vi "Smile_Or_Frown.vi"() -> (0 "New Values In":string[][](array[string])=[["Test data5"]], 1 "New Chs In":string[](array[string])=["30-10-03:New:Channel new5"])   [LabVIEW 2022 SP3]
uses:
  <vilib>/Analysis/baseanly.llb/Mean (DBL).vi
  Results_plotter_Global.vi
  Data plotting/subVIs/Plot_Values_Global.vi
  <vilib>/Analysis/NI_AALBase.lvlib
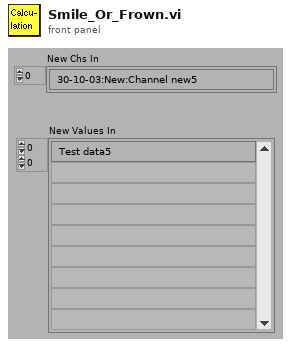
[diagram p1: front panel]
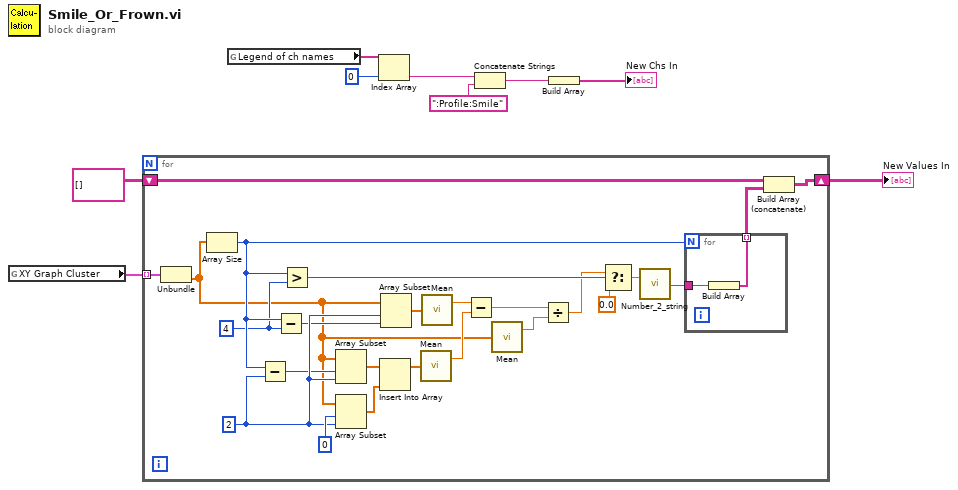
[diagram p0: block diagram]
diagram:
  n1 = global read "Plot_Values_Global.vi" "XY Graph Cluster"() -> (w1:cluster{dbl[], dbl[]}[])
  n2 = for {
    tunnel: w1 -> [w33] mode=indexing
    shift-right: [w30] -> w5
    shift-left: string[][] [] -> [w32]
    w22 = 2 ("length")
    w16 = 4 ("y")
    n3 = Unbundle(w33) -> (w13:dbl[])  [unwired: 1 out]
    n4 = Array Size(array=w13) -> (size(s)=w17:i32)
    n5 = Subtract(x=w17, y=w22) -> (x-y=w15:i32)
    n6 = Subtract(x=w17, y=w16) -> (x-y=w14:i32)
    n7 = Greater?(x=w17, y=w16) -> (0:w20:bool)
    n8 = Array Subset(array=w13, index=w15, length=w22) -> (w27:dbl[])
    n9 = Array Subset(array=w13, index=0, length=w22) -> (w26:dbl[])
    n10 = Insert Into Array(array=w27, new element=w26) -> (w25:dbl[])  [unwired: 1 in]
    n11 = Array Subset(array=w13, index=w22, length=w14) -> (w21:dbl[])
    n12 = call-poly <vilib>:"Mean.vi"("X"=w25) -> ("mean"=w23:dbl)  [unwired: 1 out]
    n13 = call-poly <vilib>:"Mean.vi"("X"=w21) -> ("mean"=w24:dbl)  [unwired: 1 out]
    n14 = Subtract(x=w24, y=w23) -> (x-y=w11:dbl)
    n15 = call-poly <vilib>:"Mean.vi"("X"=w13) -> ("mean"=w12:dbl)  [unwired: 1 out]
    n16 = Divide(x=w11, y=w12) -> (x/y=w10:dbl)
    n17 = Select(t=w10, s=w20, f=0.0) -> (s? t:f=w18:dbl)
    n18 = call "Number_2_string.vi"("number"=w18) -> ("String"=w29:string)  [unwired: 1 in]
    n19 = for {
      N: w17 -> [_]
      tunnel: [w35] -> w31 mode=indexing
      tunnel: w29 -> [w34]
      n20 = Build Array(w34) -> (w35:string[])
    }
    n21 = Build Array (concatenate)(w32, w31) -> (w30:string[][])
  }
  "New Values In" <- w5
  n22 = global read "Results_plotter_Global.vi" "Legend of ch names"() -> (w7:string[])
  n23 = Index Array(array=w7, index=0) -> (element=w3:string)
  n24 = Concatenate Strings(w3, ":Profile:Smile" ("string")) -> (w2:string)
  n25 = Build Array(w2) -> (→"New Chs In":string[])
